vi "oef14.7.vi"() -> ()   [LabVIEW 2021]
uses:
  <vilib>/express/express arith-compare/Formula/XNode/ExpressFormulaBlockNode.xnode
panel:
  in  "stop":bool
  out "Waveform Graph":dbl[](graph)
  in  "R":dbl(knob) scale=0.0..100.0
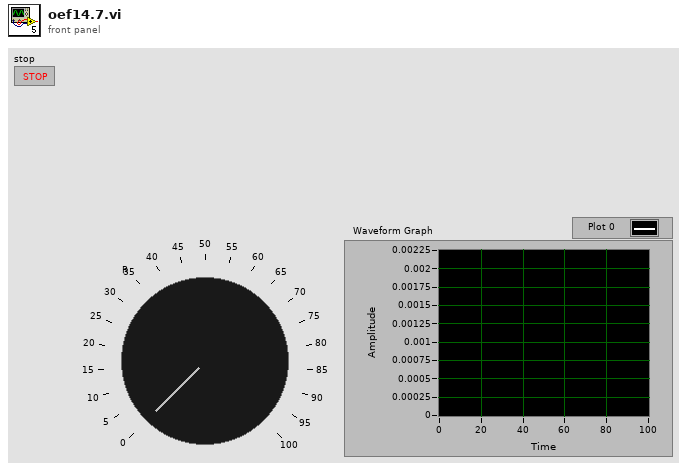
[diagram p1: front panel]
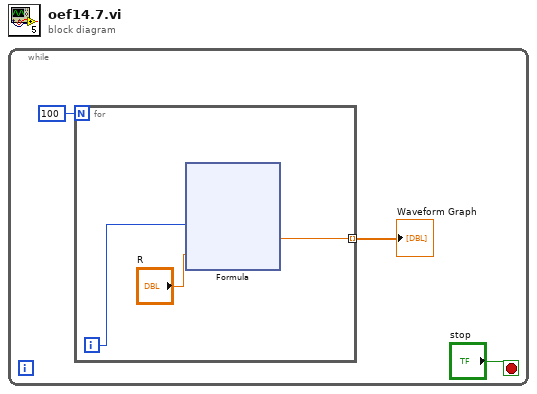
[diagram p0: block diagram]
diagram:
  n1 = while {
    stop <- "stop" stop-if-true
    n2 = for {
      N: 100 -> [_]
      tunnel: [w4] -> w2 mode=indexing
      i -> [w5]
      n3 = xnode "Formula"("C1"=w5, "R"="R") -> ("Result"=w4:dbl)  [unwired: 1 in, 1 out]
    }
    "Waveform Graph" <- w2
  }
